vi "Initdrv.vi"() -> ()   [LabVIEW 2015]
uses:
  lwlscdll.dll
panel:
  out "Numerisch":dbl format="%.2f"
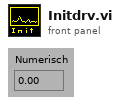
[diagram p1: front panel]
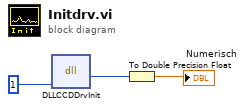
[diagram p0: block diagram]
diagram:
  n1 = dll-call lib="G:/SD/IR-det/lv/2cam/board.vis/lwlscdll.dll" fn="DLLCCDDrvInit"("drv"=u32 1) -> ("Rückgabetyp"=w3:u8)  [unwired: 4 in, 2 out]
  n2 = To Double Precision Float(number=w3) -> (double precision float=→"Numerisch":dbl)
